vi "myRIO_BRig_Host_TCP_parseCmd_selectResponse.vi"(10 "input_countCmd":i32, 11 "input_strCmd":string) -> (2 "output_selectResponse_num":i32, 3 "output_selectResponse_str":string)   [LabVIEW 2014]
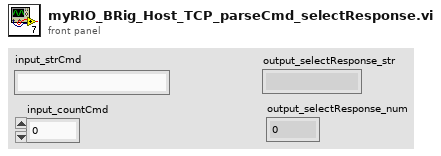
[diagram p1: front panel]
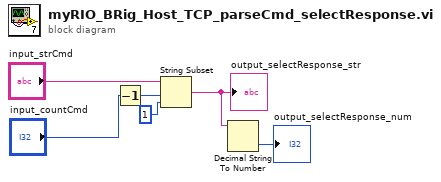
[diagram p0: block diagram]
diagram:
  n1 = Decrement(x="input_countCmd") -> (x-1=w4:i32)
  n2 = String Subset(string="input_strCmd", offset (0)=w4, length (rest)=1 ("length (rest)")) -> (substring=w5:string)
  "output_selectResponse_str" <- w5
  n3 = Decimal String To Number(string=w5) -> (number=→"output_selectResponse_num":i32)  [unwired: 2 in, 1 out]
